vi "WriteConfig.vi"(8 "error in (no error)":errorcluster, 10 "Config":variant, 11 "Sim_Ideal_PMU in":refnum<class "Sim_Ideal_PMU.lvclass">) -> (0 "error out":errorcluster, 3 "Sim_Ideal_PMU out":refnum<class "Sim_Ideal_PMU.lvclass">)   [LabVIEW 2018, in "SensorPlugins.lvlib" / "Sim_Ideal_PMU.lvclass"]
uses:
  Sim_Ideal_PMU.lvclass
  PmuBaseClass/PmuBase.lvclass
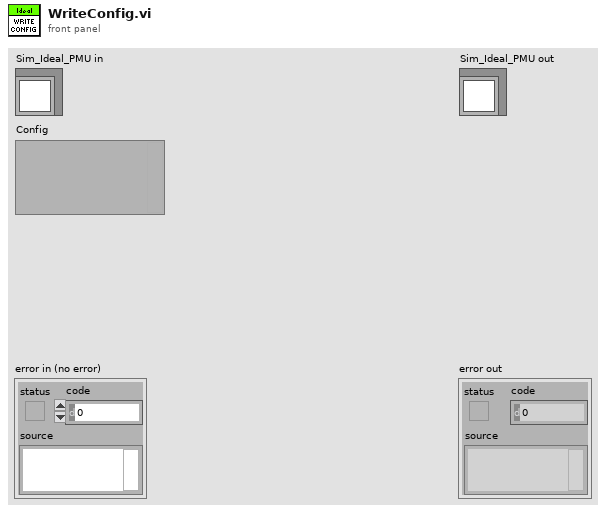
[diagram p1: front panel]
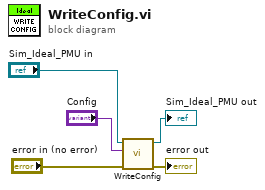
[diagram p0: block diagram]
diagram:
  n1 = call-parent "WriteConfig.vi"("error in (no error)"="error in (no error)", "Config"="Config", "PmuBase in"="Sim_Ideal_PMU in") -> ("error out"=→"error out":errorcluster, "PmuBase out"=→"Sim_Ideal_PMU out":refnum<class "Sim_Ideal_PMU.lvclass">)  [unwired: 7 in]
